vi "HMI PopUP KB.vi"(4 "Password Display (F)":bool, 5 "Hide OVR Key (T)":bool, 6 "Max Length (70)":i32=70, 10 "String In":string, 11 "Message In":string) -> (1 "Canceled":bool, 2 "String Out":string)   [LabVIEW 2010]
doc: "Name: Pop Up Keyboard\n\nDESCRIPTION\nSimulates an alphanumeric keyboard intended to be used on a touchscreen PC. The input control can be set for standard or password display. The OVR key can be shown or hidden.\n\nINPUTS\nMessage In - Optional message displayedin the title bar.\nString In - Sets the initial value of the edit box.\nPassword Display (F) - Sets standard or password display.\nHide OVR Key (T) - Hides or displays the OVR key button.\nMax Length (255) - Sets the maximum length allowed in the edit box.\n\nOUTPUTS\nString Out - Result (will contain String In if the user cancels).\nCanceled - True if the user cancels.\n\n----------------------------------------------------------------------------------------------------------------"
uses:
  HMI PopUp KB.llb/Driver Commands.ctl
panel:
  in  "ENTER":bool
  out "Caps on":bool
  in  "Shift 2":bool
  in  "<\n,":bool
  in  "?\n/":bool
  in  ">\n.":bool
  in  "M\nm":bool
  in  "N\nn":bool
  in  "B\nb":bool
  in  "V\nv":bool
  in  "C\nc":bool
  in  "X\nx":bool
  in  "Z\nz":bool
  in  "\"\n'":bool
  in  ":\n;":bool
  in  "L\nl":bool
  in  "K\nk":bool
  in  "J\nj":bool
  in  "H\nh":bool
  in  "G\ng":bool
  in  "F\nf":bool
  in  "D\nd":bool
  in  "S\ns":bool
  in  "A\na":bool
  in  "}\n]":bool
  in  "{\n[":bool
  in  "|\n\\":bool
  in  "+\n=":bool
  in  "_\n-":bool
  in  "P\np":bool
  in  "O\no":bool
  in  "I\ni":bool
  in  "U\nu":bool
  in  "Y\ny":bool
  in  "T\nt":bool
  in  "R\nr":bool
  in  "E\ne":bool
  in  "W\nw":bool
  in  ")\n0":bool
  in  "(\n9":bool
  in  "*\n8":bool
  in  "&\n7":bool
  in  "^\n6":bool
  in  "%\n5":bool
  in  "$\n4":bool
  in  "#\n3":bool
  in  "@\n2":bool
  in  "!\n1":bool
  in  "Q\nq":bool
  in  "Right":bool
  in  "Left":bool
  in  "Over Write":bool
  in  "Ok":bool
  in  "Cancel":bool
  in  "Space":bool
  in  "Shift":bool
  in  "CAPS":bool
  in  "Text":string
  in  "Backspace":bool
  # "Inputs"
  # "Outputs"
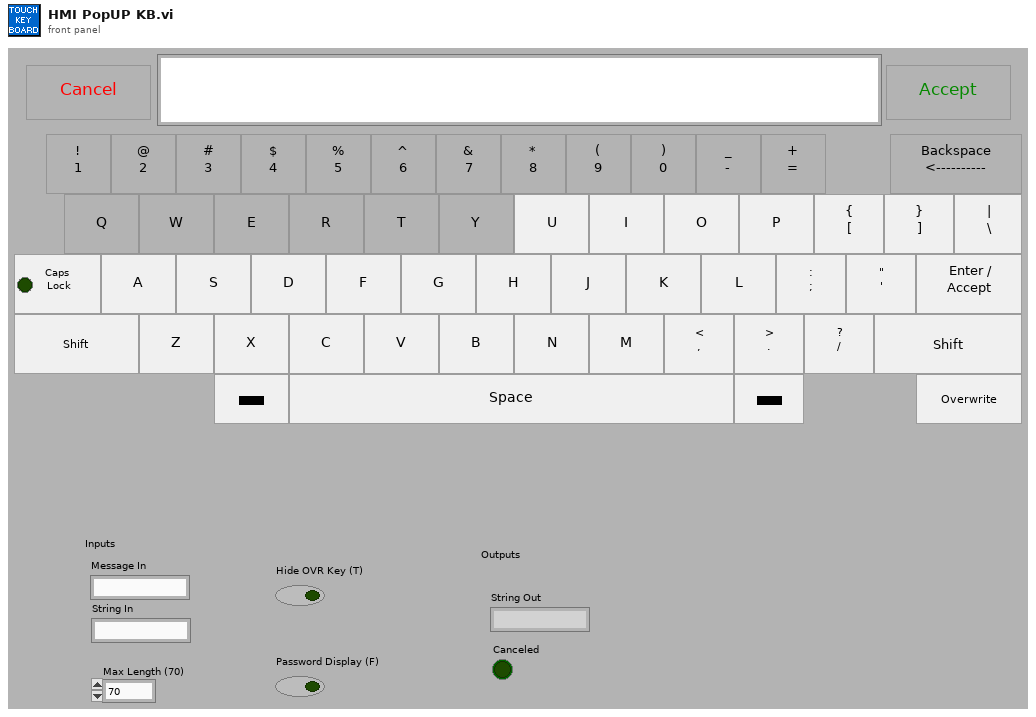
[diagram p1: front panel]
types:
  T1 = typedef "Driver Commands.ctl" = enum16{"No Command", "Initialize", "Add Character", "Replace Charcter", "Delete Character", "Move Left", "Move Right", "Update Edit Position"}
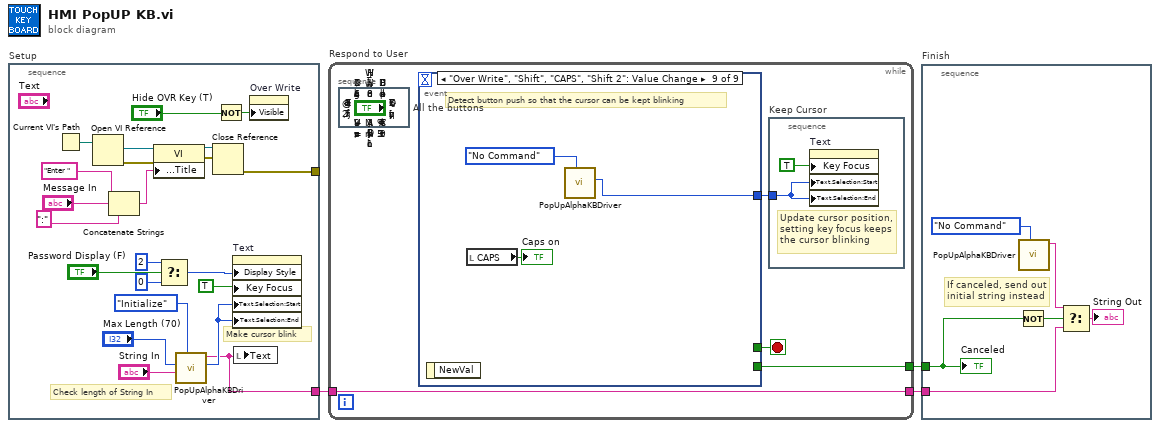
[diagram p0: block diagram]
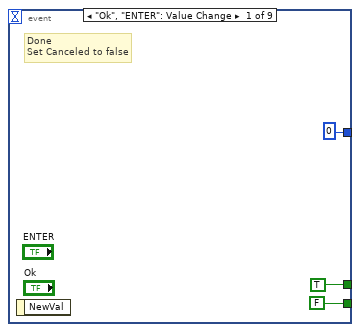
[diagram p2: hidden frame]
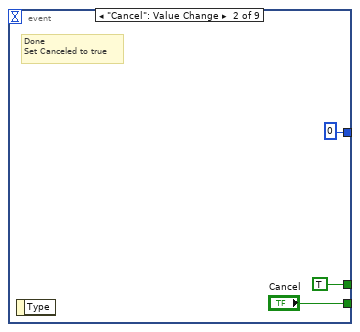
[diagram p3: hidden frame]
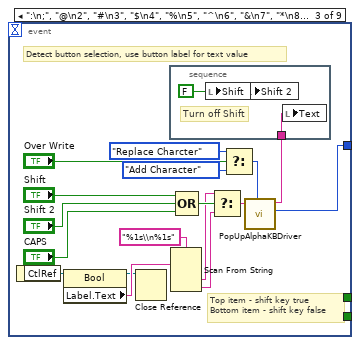
[diagram p4: hidden frame]
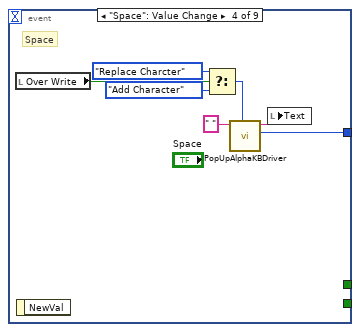
[diagram p5: hidden frame]
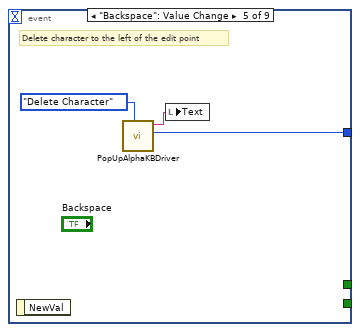
[diagram p6: hidden frame]
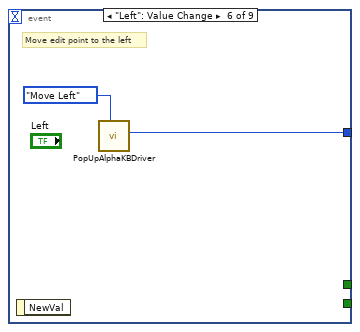
[diagram p7: hidden frame]
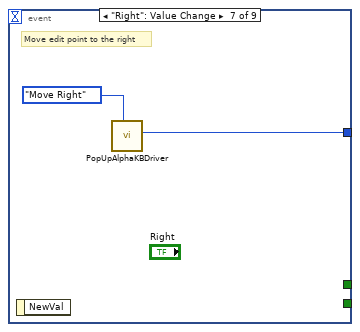
[diagram p8: hidden frame]
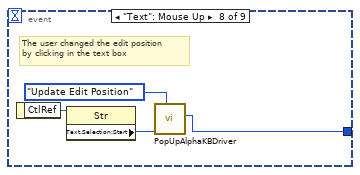
[diagram p9: hidden frame]
diagram:
  n1 = stacked-sequence "Setup" {
    tunnel: [w15] -> w3
    tunnel: [w4] -> _
    frame #0 {
      # "Make cursor blink"
      # "Check length of String In"
      n2 = Current VI's Path() -> (path=w8:path)
      n3 = Open VI Reference(vi path=w8) -> (vi reference=w9:refnum<vi>, error out=w10:errorcluster)  [unwired: 1 in, 4 out]
      n4 = Concatenate Strings("Enter ", "Message In", ":" ("Substring")) -> (w13:string)
      n5 = property class="VI"(reference=w9, error in=w10, "Front Panel Window:Title"=w13) -> (reference out=w11:refnum<vi>, error out=w12:errorcluster)
      n6 = Select(t=u32 2 ("Display Style"), s="Password Display (F)", f=u32 0 ("Display Style")) -> (s? t:f=w19:u32)
      n7 = call "PopUpAlphaKBDriver.vi"("Driver Commands"=Driver_Commands."Initialize", "Initial String"="String In", "Max Length (70)"="Max Length (70)") -> ("Edit Position"=w16:i32, "String Out"=w15:string)  [unwired: 2 in, 5 out]
      n8 = Close Reference(reference=w11, error in (no error)=w12) -> (error out=w4:errorcluster)
      n9 = Not(x="Hide OVR Key (T)") -> (.not. x?=w21:bool)
      n10 = property on="Text" class="Str"("Display Style"=w19, "Key Focus"=TRUE, "Text.Selection:Start"=w16, "Text.Selection:End"=w16) -> ()  [unwired: 2 in, 2 out]
      n11 = local write "Text"(w15) -> ()
      n12 = property on="Over Write" class="Bool (strict)"("Visible"=w21) -> ()  [unwired: 2 in, 2 out]
    }
  }
  n13 = while "Respond to User" {
    tunnel: w3 -> [w26]
    tunnel: [w27] -> w2
    tunnel: [w26] -> w1
    stop <- w29 stop-if-true
    n14 = stacked-sequence "All the buttons" {
      frame #0 {
      }
    }
    n15 = event shown="[8] \"Over Write\", \"Shift\", \"CAPS\", \"Shift 2\": Value Change" {
      selector: _ -> [_ _ _ _ _ _ _ _ _]
      dyn-events: _ -> [_ _ _ _ _ _ _ _ _]
      timeout: _ -> [_ _ _ _ _ _ _ _ _]
      tunnel: [TRUE TRUE _ _ _ _ _ _ _] -> w29
      tunnel: [0 ("Edit Position") 0 ("Edit Position") w43 w59 w65 w68 w69 w71 w76] -> w28
      tunnel: [FALSE ("Cancel") "Cancel" _ _ _ _ _ _ _] -> w27
      event "Ok", "ENTER": Value Change {
        # "Done\nSet Canceled to false"
        n16 = event-data() -> ()  [unwired: 2 out]
      }
      event "Cancel": Value Change {
        # "Done\nSet Canceled to true"
        n17 = event-data() -> ()  [unwired: 2 out]
      }
      event ":\n;", "@\n2", "#\n3", "$\n4", "%\n5", "^\n6", "&\n7", "*\n8", "(\n9", ")\n0", "_\n-", "+\n=", "|\n\\", "Q\nq", "W\nw", "E\ne", "R\nr", "T\nt", "Y\ny", "U\nu", "I\ni", "O\no", "P\np", "A\na", "S\ns", "D\nd", "F\nf", "G\ng", "H\nh", "J\nj", "K\nk", "L\nl", "\"\n'", "Z\nz", "X\nx", "C\nc", "V\nv", "B\nb", "N\nn", "M\nm", "<\n,", ">\n.", "?\n/", "}\n]", "!\n1": Value Change {
        # "Top item - shift key true\nBottom item - shift key false"
        # "Detect button selection, use button label for text value"
        n18 = event-data() -> ("CtlRef"=w50:refnum<vi>)  [unwired: 1 out]
        n19 = property class="Bool"(reference=w50) -> (reference out=w48:refnum<vi>, "Label.Text"=w49:string)  [unwired: 1 in, 1 out]
        n20 = Close Reference(reference=w48) -> ()  [unwired: 1 in, 1 out]
        n21 = Scan From String(format string="%1s\\n%1s", input string=w49) -> (output 1=w52:string, output 2=w51:string)  [unwired: 2 in, 5 out]
        n22 = Compound Arithmetic op=OR("Shift", "Shift 2", "CAPS") -> (w53:bool)
        n23 = Select(t=w52, s=w53, f=w51) -> (s? t:f=w47:string)
        n24 = Select(t=Driver_Commands."Replace Charcter" ("Driver Commands"), s="Over Write", f=Driver_Commands."Add Character" ("Driver Commands")) -> (s? t:f=w46:T1)
        n25 = call "PopUpAlphaKBDriver.vi"("Driver Commands"=w46, "Character"=w47) -> ("Edit Position"=w43:i32, "String Out"=w41:string)  [unwired: 3 in, 5 out]
        n26 = stacked-sequence {
          tunnel: w41 -> [w56]
          frame #0 {
            w55 = FALSE ("Shift")
            # "Turn off Shift"
            n27 = local write "Shift"(w55) -> ()
            n28 = local write "Shift 2"(w55) -> ()
            n29 = local write "Text"(w56) -> ()
          }
        }
      }
      event "Space": Value Change {
        # "Space"
        n30 = local read "Over Write"() -> (w57:bool)
        n31 = event-data() -> ()  [unwired: 2 out]
        n32 = Select(t=Driver_Commands."Replace Charcter" ("Driver Commands"), s=w57, f=Driver_Commands."Add Character" ("Driver Commands")) -> (s? t:f=w60:T1)
        n33 = call "PopUpAlphaKBDriver.vi"("Driver Commands"=w60, "Character"=" ") -> ("Edit Position"=w59:i32, "String Out"=w58:string)  [unwired: 3 in, 5 out]
        n34 = local write "Text"(w58) -> ()
      }
      event "Backspace": Value Change {
        # "Delete character to the left of the edit point"
        n35 = event-data() -> ()  [unwired: 2 out]
        n36 = call "PopUpAlphaKBDriver.vi"("Driver Commands"=Driver_Commands."Delete Character") -> ("Edit Position"=w65:i32, "String Out"=w64:string)  [unwired: 4 in, 5 out]
        n37 = local write "Text"(w64) -> ()
      }
      event "Left": Value Change {
        # "Move edit point to the left"
        n38 = event-data() -> ()  [unwired: 2 out]
        n39 = call "PopUpAlphaKBDriver.vi"("Driver Commands"=Driver_Commands."Move Left") -> ("Edit Position"=w68:i32)  [unwired: 4 in, 6 out]
      }
      event "Right": Value Change {
        # "Move edit point to the right"
        n40 = event-data() -> ()  [unwired: 2 out]
        n41 = call "PopUpAlphaKBDriver.vi"("Driver Commands"=Driver_Commands."Move Right") -> ("Edit Position"=w69:i32)  [unwired: 4 in, 6 out]
      }
      event "Text": Mouse Up {
        # "The user changed the edit position\nby clicking in the text box"
        n42 = event-data() -> ("CtlRef"=w74:refnum<vi>)  [unwired: 1 out]
        n43 = property class="Str"(reference=w74) -> ("Text.Selection:Start"=w73:u32)  [unwired: 1 in, 2 out]
        n44 = call "PopUpAlphaKBDriver.vi"("Driver Commands"=Driver_Commands."Update Edit Position", "New Edit Position"=w73) -> ("Edit Position"=w71:i32)  [unwired: 3 in, 6 out]
      }
      event "Over Write", "Shift", "CAPS", "Shift 2": Value Change {
        # "Detect button push so that the cursor can be kept blinking"
        n45 = event-data() -> ()  [unwired: 2 out]
        n46 = local read "CAPS"() -> (→"Caps on":bool)
        n47 = call "PopUpAlphaKBDriver.vi"("Driver Commands"=Driver_Commands."No Command") -> ("Edit Position"=w76:i32)  [unwired: 4 in, 6 out]
      }
    }
    n48 = stacked-sequence "Keep Cursor" {
      tunnel: w28 -> [w30]
      frame #0 {
        # "Update cursor position,\nsetting key focus keeps\nthe cursor blinking"
        n49 = property on="Text" class="Str"("Key Focus"=TRUE, "Text.Selection:Start"=w30, "Text.Selection:End"=w30) -> ()  [unwired: 2 in, 2 out]
      }
    }
  }
  n50 = stacked-sequence "Finish" {
    tunnel: w2 -> [w82]
    tunnel: w1 -> [w79]
    frame #0 {
      # "If canceled, send out\ninitial string instead"
      n51 = Not(x=w82) -> (.not. x?=w80:bool)
      n52 = call "PopUpAlphaKBDriver.vi"("Driver Commands"=Driver_Commands."No Command") -> ("String Out"=w78:string)  [unwired: 4 in, 6 out]
      n53 = Select(t=w78, s=w80, f=w79) -> (s? t:f=→"String Out":string)
      "Canceled" <- w82
    }
  }
